vi "Write.vi"(10 "String Array":timestamp[](array[timestamp]), 11 "String Array in":refnum<class "Time Stamp Array.lvclass">) -> (3 "String Array out":refnum<class "Time Stamp Array.lvclass">)   [LabVIEW 2020, in "Data.lvlib" / "Time Stamp Array.lvclass"]
doc: "Write Time Stamp Array."
uses:
  Time Stamp Array.lvclass
  Time Stamp Array.lvclass/Time Stamp Array.ctl
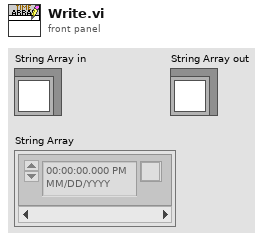
[diagram p1: front panel]
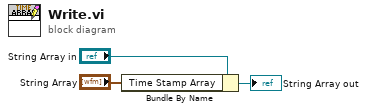
[diagram p0: block diagram]
diagram:
  n1 = Bundle By Name(cluster="String Array in", "Time Stamp Array"="String Array") -> (→"String Array out":refnum<class "Time Stamp Array.lvclass">)
